vi "文件写入.vi"() -> ()   [LabVIEW 2021]
uses:
  <vilib>/Utility/file.llb/Write Delimited Spreadsheet (DBL).vi
  <vilib>/Utility/file.llb/Read Delimited Spreadsheet (DBL).vi
panel:
  out "?":bool
  in  "文件名":string
  in  "?":string[][](table)
  in  "?":bool
  in  "?":bool
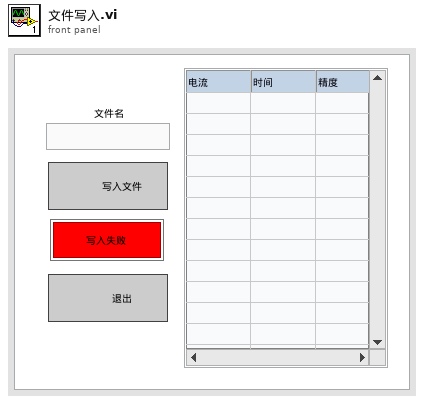
[diagram p1: front panel]
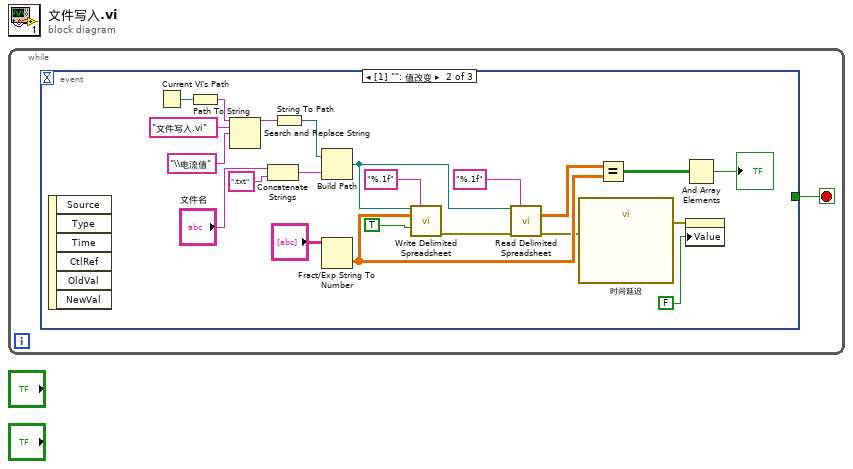
[diagram p0: block diagram]
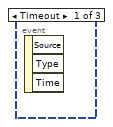
[diagram p2: hidden frame]
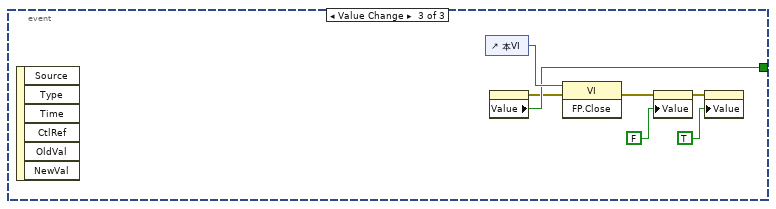
[diagram p3: hidden frame]
diagram:
  n1 = while {
    stop <- w1 stop-if-true
    n2 = event shown="[1] \"\": 值改变" {
      selector: _ -> [_ _ _]
      dyn-events: _ -> [_ _ _]
      timeout: _ -> [_ _ _]
      tunnel: [_ _ w27] -> w1
      event Timeout {
        n3 = event-data() -> ()  [unwired: 1 in, 3 out]
      }
      event Value Change {
        n4 = event-data() -> ()  [unwired: 1 in, 6 out]
        n5 = Current VI's Path() -> (path=w6:path)
        n6 = Path To String(path=w6) -> (string=w4:string)
        n7 = Search and Replace String(input string=w4, search string="文件写入.vi" ("搜索字符串"), replace string="\\电流值" ("字符串")) -> (result string=w2:string)  [unwired: 5 in, 3 out]
        n8 = Concatenate Strings("文件名", ".txt" ("字符串")) -> (w21:string)
        n9 = String To Path(string=w2) -> (path=w7:path)
        n10 = Build Path(base path=w7, name or relative path=w21) -> (appended path=w16:path)
        n11 = Fract/Exp String To Number(string="?") -> (number=w14:dbl[][])  [unwired: 3 in, 1 out]
        n12 = call-poly <vilib>:"Write Delimited Spreadsheet.vi"("file path (dialog if empty)"=w16, "format (%.3f)"="%.1f", "2D data"=w14, "append to file? (new file:F)"=TRUE) -> ("error out"=w17:errorcluster)  [unwired: 10 in, 1 out]
        n13 = call-poly <vilib>:"Read Delimited Spreadsheet.vi"("file path (dialog if empty)"=w16, "format (%.3f)"="%.1f", "error in (no error)"=w17) -> ("all rows"=w15:dbl[][], "error out"=w9:errorcluster)  [unwired: 7 in, 4 out]
        n14 = call "时间延迟"("error in (no error)"=w9) -> ("error out"=w8:errorcluster)  [unwired: 10 in]
        n15 = Equal?(x=w15, y=w14) -> (x = y?=w12:bool[][])
        n16 = And Array Elements(Boolean array=w12) -> (logical AND=→"?":bool)
        n17 = property class="Bool (严格)"(error in=w8, "Value"=FALSE) -> ()  [unwired: 1 in, 2 out]
      }
      event Value Change {
        n18 = event-data() -> ()  [unwired: 1 in, 6 out]
        n19 = control-ref of="本VI"() -> (w30:refnum<vi>)
        n20 = property class="Bool (严格)"() -> (error out=w26:errorcluster, "Value"=w27:bool)  [unwired: 2 in, 1 out]
        n21 = invoke class="VI" method="FP.Close"(reference=w30, error in=w26) -> (error out=w29:errorcluster)  [unwired: 1 in, 2 out]
        n22 = property class="Bool (严格)"(error in=w29, "Value"=FALSE) -> (error out=w25:errorcluster)  [unwired: 1 in, 1 out]
        n23 = property class="Bool (严格)"(error in=w25, "Value"=TRUE) -> ()  [unwired: 1 in, 2 out]
      }
    }
  }
